vi "Disconnect.vi"(8 "error in (no error)":errorcluster, 11 "TektronixDPO_PhysicalDevice in":refnum<class "TektronixDPO_PhysicalDevice.lvclass">) -> (0 "error out":errorcluster)   [LabVIEW 2013, in "TektronixDPO_PhysicalDevice.lvclass"]
uses:
  TektronixDPO_PhysicalDevice.lvclass
  TektronixDPO_PhysicalDevice.lvclass/TektronixDPO_PhysicalDevice.ctl
  Tektronix DPO MSO 2000 4000 Series/Tektronix DPO MSO 2000 4000 Series.lvlib
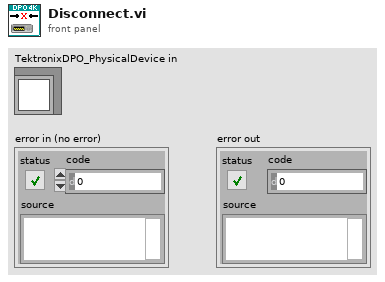
[diagram p1: front panel]
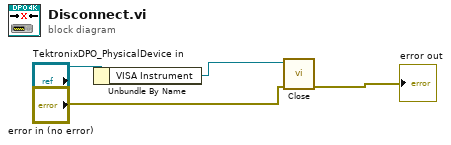
[diagram p0: block diagram]
diagram:
  n1 = Unbundle By Name("TektronixDPO_PhysicalDevice in") -> ("VISA Instrument"=w2:refnum<visa-resource-name>)
  n2 = call "Close.vi"("error in (no error)"="error in (no error)", "VISA resource name"=w2) -> ("error out"=→"error out":errorcluster)  [unwired: 9 in]
